vi "Auto_Routine_Deposit_Backup_Balance.vi"(8 "error in (no error)":errorcluster) -> (0 "error out":errorcluster)   [LabVIEW 2020]
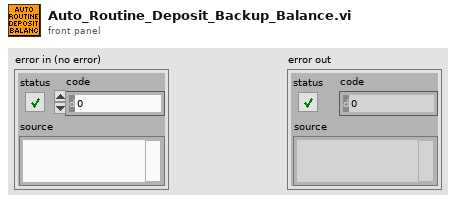
[diagram p1: front panel]
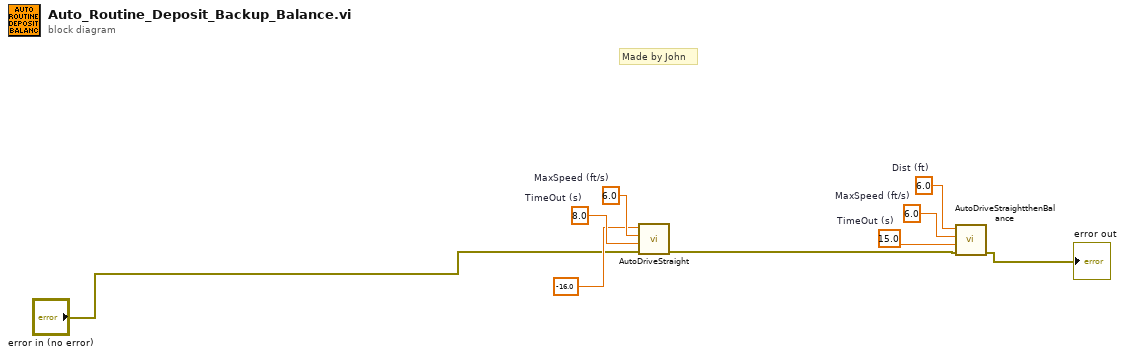
[diagram p0: block diagram]
diagram:
  w4 = 15.0  # TimeOut (s)
  w5 = 6.0  # MaxSpeed (ft/s)
  w6 = 6.0  # Dist (ft)
  w7 = 8.0  # TimeOut (s)
  w8 = 6.0  # MaxSpeed (ft/s)
  # "Made by John"
  n1 = call "AutoDriveStraight.vi"("error in (no error)"="error in (no error)", "TimeOut (s)"=w7, "MaxSpeed (ft/s)"=w8, "Dist (ft)"=-16.0) -> ("error out"=w9:errorcluster)  [unwired: 7 in]
  n2 = call "AutoDriveStraightthenBalance.vi"("error in (no error)"=w9, "TimeOut (s)"=w4, "MaxSpeed (ft/s)"=w5, "Dist (ft)"=w6) -> ("error out"=→"error out":errorcluster)  [unwired: 7 in]
